vi "Close.vi"(8 "error in (no error)":errorcluster, 11 "Measurement3D in":refnum<class "Measurement3D.lvclass">) -> (0 "error out":errorcluster, 3 "Measurement3D out":refnum<class "Measurement3D.lvclass">)   [LabVIEW 2014, in "Measurement3D.lvclass"]
uses:
  Measurement3D.lvclass
  Instrument/Instrument/Instrument.lvclass
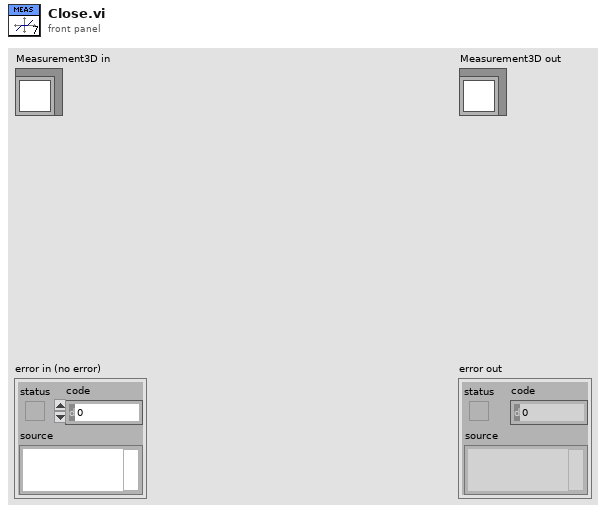
[diagram p1: front panel]
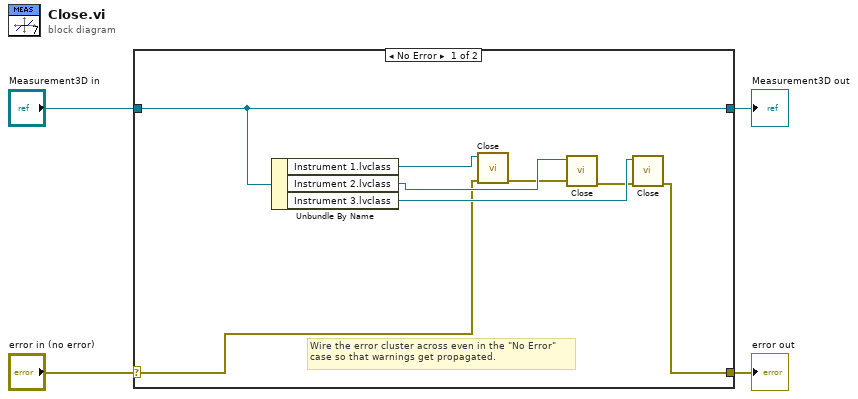
[diagram p0: block diagram]
diagram:
  n1 = case shown="No Error" "error in (no error)" {
    selector: "error in (no error)" -> [w6 w14]
    tunnel: [w5 w14] -> w3
    tunnel: [w9 w13] -> w1
    tunnel: "Measurement3D in" -> [w9 w13]
    frame No Error {
      # "Wire the error cluster across even in the \"No Error\"\ncase so that warnings get propagated."
      n2 = Unbundle By Name(w9) -> ("Instrument 1.lvclass"=w12:refnum<class "Instrument.lvclass">, "Instrument 2.lvclass"=w11:refnum<class "Instrument.lvclass">, "Instrument 3.lvclass"=w8:refnum<class "Instrument.lvclass">)
      n3 = call-dynamic "Close.vi"("error in (no error)"=w6, "Instrument in"=w12) -> ("error out"=w10:errorcluster)  [unwired: 8 in, 1 out]
      n4 = call-dynamic "Close.vi"("error in (no error)"=w10, "Instrument in"=w11) -> ("error out"=w7:errorcluster)  [unwired: 8 in, 1 out]
      n5 = call-dynamic "Close.vi"("error in (no error)"=w7, "Instrument in"=w8) -> ("error out"=w5:errorcluster)  [unwired: 8 in, 1 out]
    }
    frame Error {
    }
  }
  "error out" <- w3
  "Measurement3D out" <- w1
